vi "Simulation.vi"() -> ()   [LabVIEW 2026]
panel:
  out "Output size":i32
  out "size(s)":i32
  out "Input bits":dbl[](array[numeric])
  out "output bits graph":dbl[](graph)
  out "Output bits":dbl[](array[numeric])
  out "Constellation graph":cluster{"Y":dbl[], "Y":dbl[]}[](graph)
  out "Input Graph":dbl[](graph)
  out "Transmitted Signal":waveform(dbl)(graph)
  in  "standard deviation":dbl=1.0000000000000002 format="%0.2f"
  in  "Sequence Size":i32
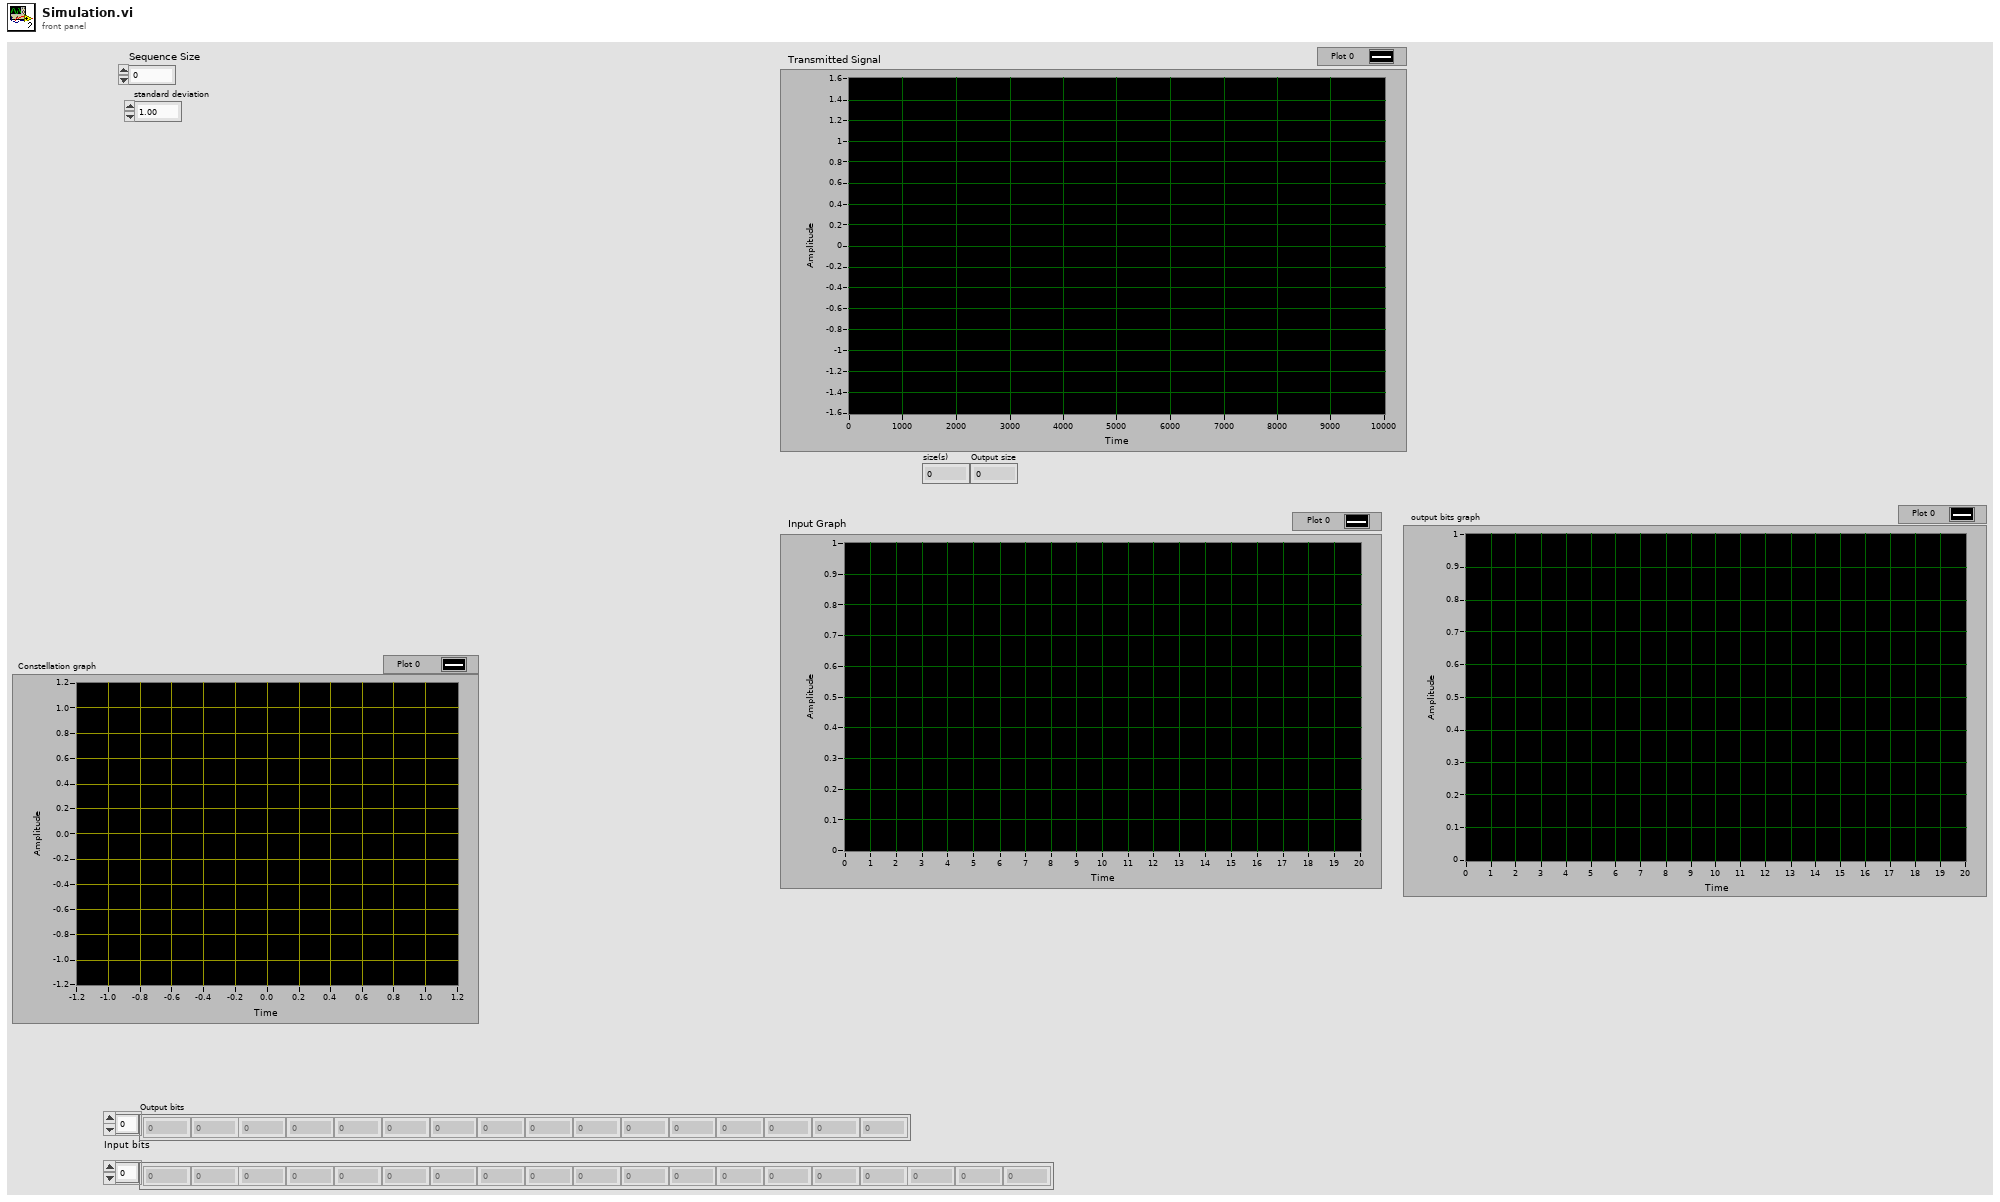
[diagram p1: front panel]
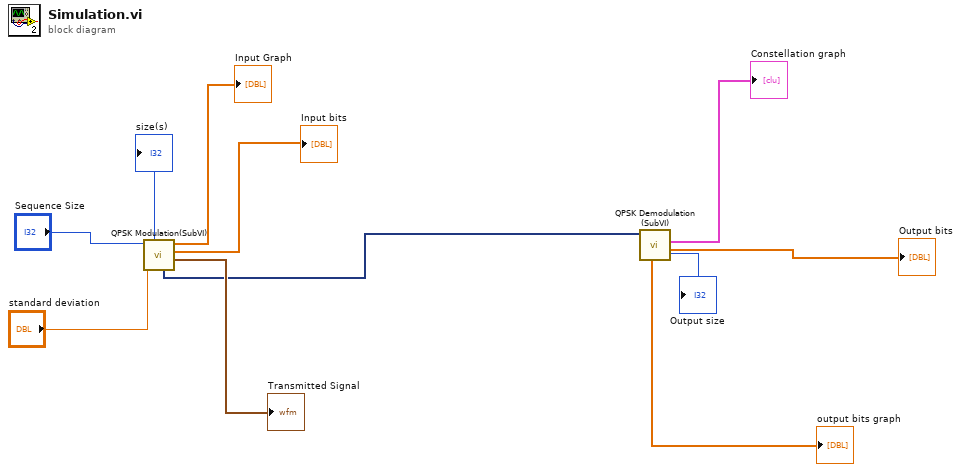
[diagram p0: block diagram]
diagram:
  n1 = call "QPSK Modulation(SubVI).vi"("standard deviation"="standard deviation", "Sequence Size"="Sequence Size") -> ("Transmitted Signal"=→"Transmitted Signal":waveform(dbl), "input bits"=→"Input bits":dbl[], "Input Graph"=→"Input Graph":dbl[], "Array"=w4:dynamicdata[], "size(s)"=→"size(s)":i32)  [unwired: 5 in]
  n2 = call "QPSK Demodulation (SubVI).vi"("Array in"=w4) -> ("Output bits"=→"Output bits":dbl[], "Constellation graph"=→"Constellation graph":cluster{"Y":dbl[], "Y":dbl[]}[], "size(s)"=→"Output size":i32, "output bits graph"=→"output bits graph":dbl[])  [unwired: 5 in, 2 out]
